vi "Flag_Update.vi"(8 "error in (no error)":errorcluster, 11 "Flag":T1) -> (0 "error out":errorcluster)   [LabVIEW 2016, in "SeqProcessor.lvlib"]
uses:
  SeqProcessor.lvlib
  controls/Flag.ctl
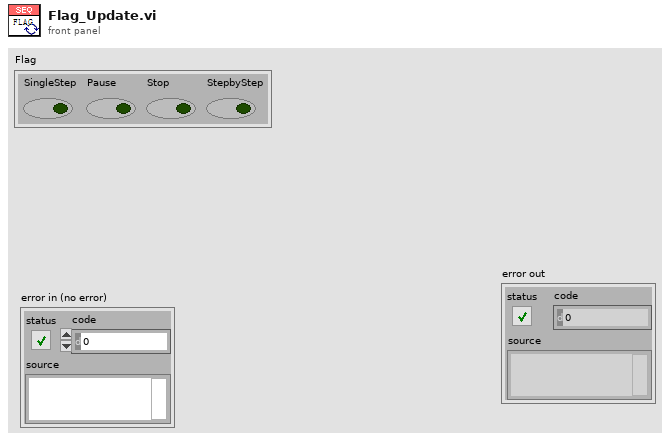
[diagram p1: front panel]
types:
  T1 = typedef "SeqProcessor.lvlib/Flag.ctl" = cluster{"SingleStep":bool, "Pause":bool, "Stop":bool, "StepbyStep":bool}
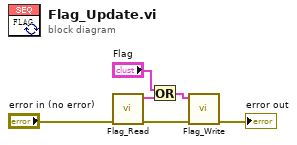
[diagram p0: block diagram]
diagram:
  n1 = call "Flag_Read.vi"("error in (no error)"="error in (no error)") -> ("error out"=w5:errorcluster, "Flag"=w3:T1)  [unwired: 8 in, 1 out]
  n2 = Or(x="Flag", y=w3) -> (x .or. y?=w2:T1)
  n3 = call "Flag_Write.vi"("error in (no error)"=w5, "Flag"=w2) -> ("error out"=→"error out":errorcluster)  [unwired: 9 in]
